vi "1553 Channels to Start and Stop Handles.vi"(8 "error in":errorcluster, 10 "1553 channels":T5[](array[typedef]), 11 "Ballard MIL-STD 1553 custom device in":T4 format="%.0x") -> (0 "error out":errorcluster, 1 "1553 start stop handles":T1[](array[typedef]) {"start stop handles"."stop handle" format="%.0x"; "start stop handles"."start handle" format="%.0x"}, 2 "start stop channels":T4[](array[typedef]) format="%.0x", 3 "Ballard MIL-STD 1553 custom device out":T4 format="%.0x")   [LabVIEW 2020, in "Ballard MIL-STD-1553 Engine.lvlib" / "Implementation.lvlib" / "Address Based Execution Unit.lvclass"]
uses:
  Address Based Execution Unit/Address Based Execution Unit.lvclass
  <vilib>/NI VeriStand/Custom Device API/Custom Device Item Ref.ctl
  <vilib>/NI VeriStand/Custom Device API/Custom Device API.lvlib
  Scripting/Ballard MIL-STD-1553 Scripting.lvlib
  Shared/Address.ctl
  Start Stop Channel Handles.ctl
  1553 Start Stop Channel Handles.ctl
  Shared/Terminal Endpoint.ctl
  Shared/Parameter Definition.ctl
  Shared/Message Type.ctl
  Shared/Message Definition.ctl
  Shared/Terminal Name and Address.ctl
  Shared/1553 Channel.ctl
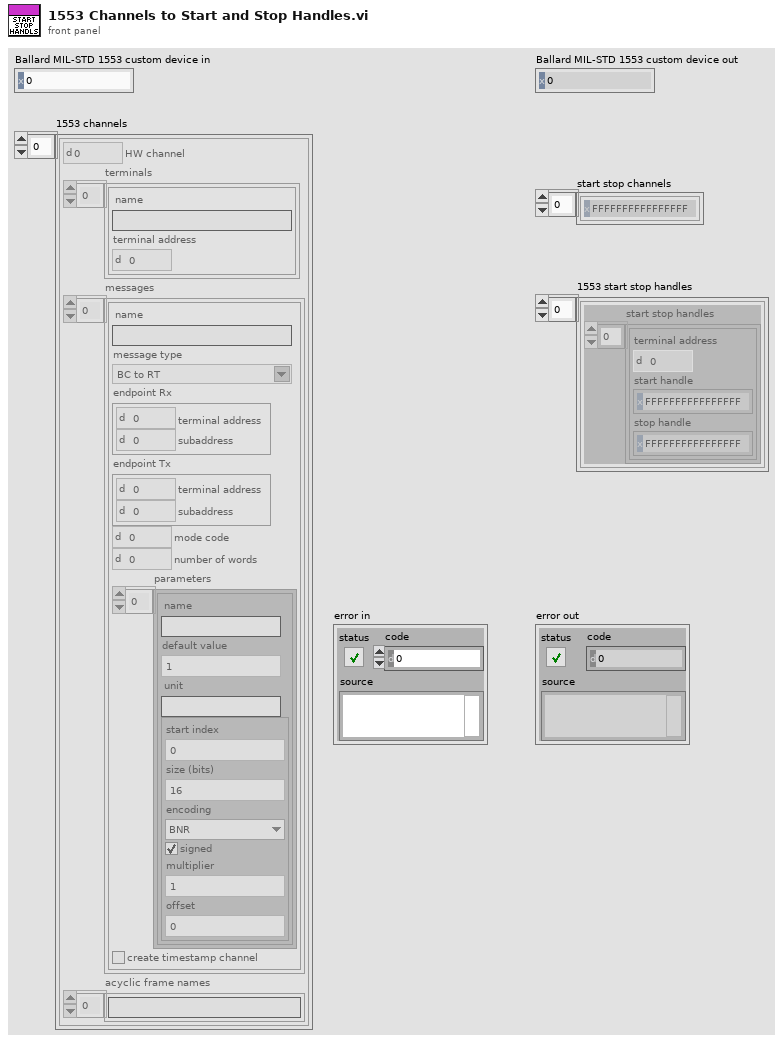
[diagram p1: front panel]
types:
  T1 = typedef "Ballard MIL-STD-1553 Engine.lvlib/Implementation.lvlib/Address Based Execution Unit.lvclass/1553 Start Stop Channel Handles.ctl" = cluster{"start stop handles":T2[]}
  T2 = typedef "Ballard MIL-STD-1553 Engine.lvlib/Implementation.lvlib/Address Based Execution Unit.lvclass/Start Stop Channel Handles.ctl" = cluster{"terminal address":T3, "start handle":T4, "stop handle":T4}
  T3 = typedef "Address.ctl" = u16
  T4 = typedef "Custom Device API.lvlib/Custom Device Item Ref.ctl" = u64
  T5 = typedef "1553 Channel.ctl" = cluster{"HW channel":u16, "terminals":T6[], "messages":T7[], "acyclic frame names":string[]}
  T6 = typedef "Terminal Name and Address.ctl" = cluster{"name":string, "terminal address":T3}
  T7 = typedef "Message Definition.ctl" = cluster{"name":string, "message type":T8, "endpoint Rx":T9, "endpoint Tx":T9, "mode code":u16, "number of words":u16, "parameters":cluster{"name":string, "default value":dbl, "unit":string, "parameter definition":T10}[], "create timestamp channel":bool}
  T8 = typedef "Message Type.ctl" = string
  T9 = typedef "Terminal Endpoint.ctl" = cluster{"terminal address":T3, "subaddress":T3}
  T10 = typedef "Parameter Definition.ctl" = cluster{"start index":i32, "size (bits)":i32, "encoding":enum16{"BNR", "BCD", "Discrete"}, "signed":bool, "multiplier":dbl, "offset":dbl}
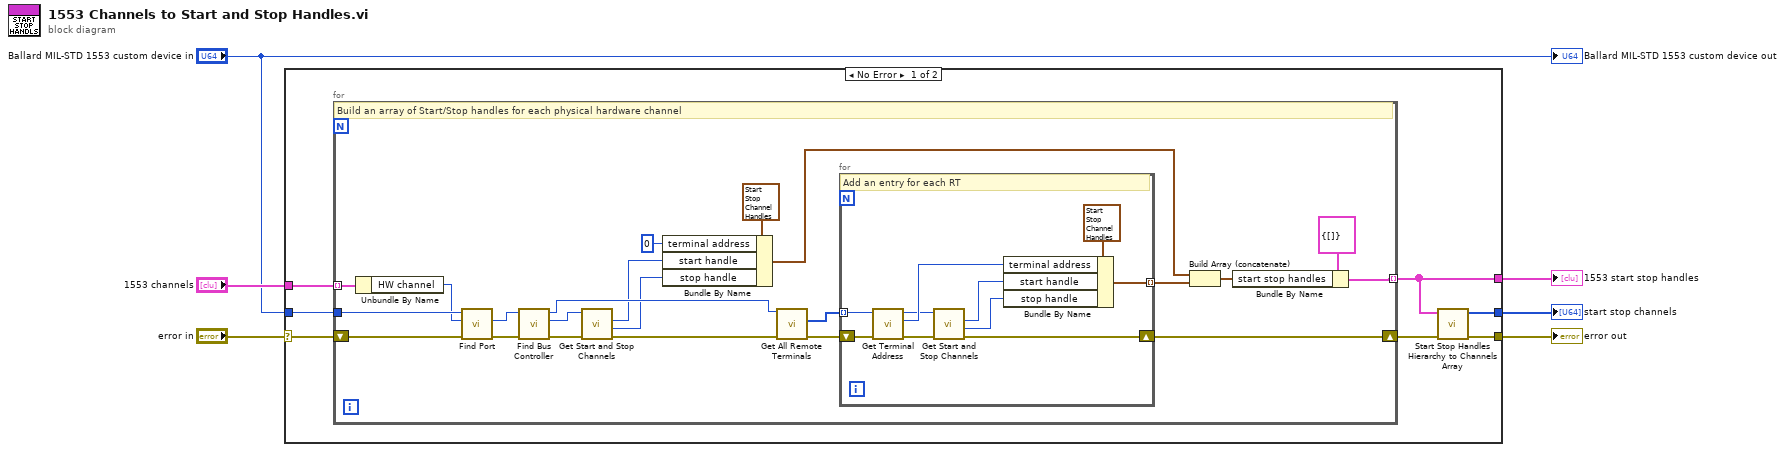
[diagram p0: block diagram]
diagram:
  n1 = case shown="No Error" "error in" {
    selector: "error in" -> [w12 w46]
    tunnel: "1553 channels" -> [w13 _]
    tunnel: "Ballard MIL-STD 1553 custom device in" -> [w11 _]
    tunnel: [w9 w46] -> w4
    tunnel: [w8 _] -> w3
    tunnel: [w7 _] -> w1
    frame No Error {
      n2 = for {
        tunnel: w13 -> [w35] mode=indexing
        shift-right: [w14] -> w10
        shift-left: w12 -> [w34]
        tunnel: w11 -> [w33]
        tunnel: [w15] -> w7 mode=indexing
        # "Build an array of Start/Stop handles for each physical hardware channel"
        n3 = Unbundle By Name(w35) -> ("HW channel"=w32:u16)
        n4 = call "Find Port.vi"("error in"=w34, "port number"=w32, "Ballard MIL-STD 1553 custom device in"=w33) -> ("error out"=w27:errorcluster, "port"=w26:T4)  [unwired: 5 in, 2 out]
        n5 = call "Find Bus Controller.vi"("error in"=w27, "port in"=w26) -> ("error out"=w29:errorcluster, "bus controller"=w28:T4, "port out"=w25:T4)  [unwired: 6 in, 1 out]
        n6 = call "Get Start and Stop Channels.vi"("error in"=w29, "terminal in"=w28) -> ("error out"=w24:errorcluster, "stop channel"=w21:T4, "start channel"=w22:T4)  [unwired: 5 in, 2 out]
        n7 = Bundle By Name(cluster=T2 {"terminal address"=0, "start handle"=18446744073709551615, "stop handle"=18446744073709551615} ("start stop handle"), "terminal address"=T3 0, "start handle"=w22, "stop handle"=w21) -> (w18:T2)
        n8 = call "Get All Remote Terminals.vi"("error in"=w24, "port in"=w25) -> ("error out"=w31:errorcluster, "remote terminals"=w30:T4[])  [unwired: 7 in, 1 out]
        n9 = for {
          shift-right: [w37] -> w14
          shift-left: w31 -> [w44]
          tunnel: w30 -> [w43] mode=indexing
          tunnel: [w36] -> w19 mode=indexing
          # "Add an entry for each RT"
          n10 = call "Get Terminal Address.vi"("error in"=w44, "remote terminal in"=w43) -> ("error out"=w41:errorcluster, "terminal address"=w42:u16, "remote terminal out"=w40:T4)  [unwired: 6 in, 1 out]
          n11 = call "Get Start and Stop Channels.vi"("error in"=w41, "terminal in"=w40) -> ("error out"=w37:errorcluster, "stop channel"=w38:T4, "start channel"=w39:T4)  [unwired: 5 in, 2 out]
          n12 = Bundle By Name(cluster=T2 {"terminal address"=0, "start handle"=18446744073709551615, "stop handle"=18446744073709551615} ("start stop handle"), "terminal address"=w42, "start handle"=w39, "stop handle"=w38) -> (w36:T2)
        }
        n13 = Build Array (concatenate)(w18, w19) -> (w16:T2[])
        n14 = Bundle By Name(cluster=T1 {"start stop handles"=[]} ("1553 start stop handles"), "start stop handles"=w16) -> (w15:T1)
      }
      n15 = call "Start Stop Handles Hierarchy to Channels Array.vi"("error in"=w10, "1553 start stop handles"=w7) -> ("error out"=w9:errorcluster, "start stop channels"=w8:T4[])  [unwired: 8 in]
    }
    frame Error {
    }
  }
  "error out" <- w4
  "start stop channels" <- w3
  "1553 start stop handles" <- w1
  "Ballard MIL-STD 1553 custom device out" <- "Ballard MIL-STD 1553 custom device in"
